vi "Load Alarm Tags and Descriptions.vi"(11 "Alarm Tag Description path":path) -> (2 "Alarm Descriptions":string[](array[string]), 3 "Alarm Array":T1[](array[typedef]))   [LabVIEW 2019]
uses:
  <userlib>/TAE/_SubVIs/TypeDefs/tae_AlarmTagConfiguration.ctl
  <vilib>/NI/Current Value Table/Compatibility/_SubVIs/TypeDefs/cvt_Data Types.ctl
  <userlib>/TAE/_SubVIs/TypeDefs/tae_AlarmConfiguration.ctl
  <userlib>/TAE/_SubVIs/TypeDefs/tae_AlarmType.ctl
  63bfb582-3dd8-4a27-9cf4-6b72469f749e.vi
  <vilib>/Array/Sort 2D Array - Pop Stack.vi
  <vilib>/Array/Sort 2D Array - Push Stack.vi
  <vilib>/Utility/file.llb/Read Delimited Spreadsheet (string).vi
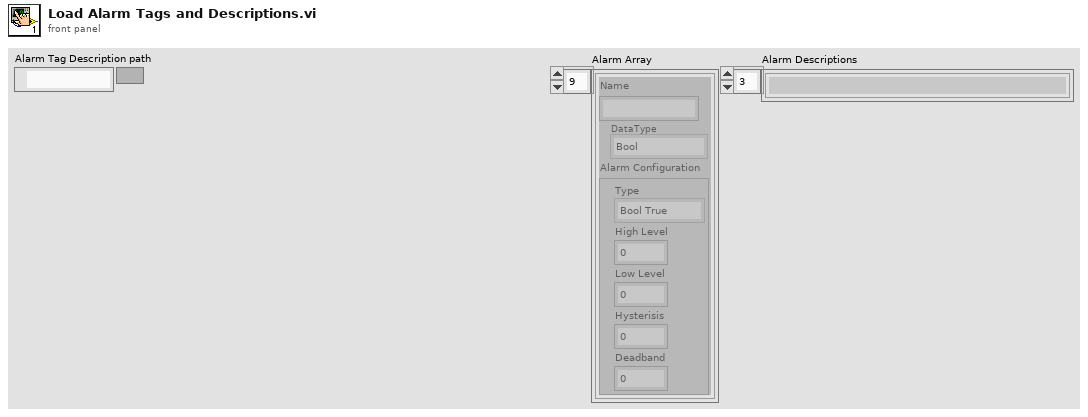
[diagram p1: front panel]
types:
  T1 = typedef "tae_AlarmTagConfiguration.ctl" = cluster{"Name":string, "DataType":T2, "Alarm Configuration":T3}
  T2 = typedef "cvt_Data Types.ctl" = enum16{"Bool", "U8", "I32", "Double", "String", "Enum"}
  T3 = typedef "tae_AlarmConfiguration.ctl" = cluster{"Type":T4, "High Level":dbl, "Low Level":dbl, "Hysterisis":dbl, "Deadband":dbl}
  T4 = typedef "tae_AlarmType.ctl" = enum32{"Bool True", "Bool False", "Over Limit", "Under Limit", "Out-of-Range", "Enum Equal", "Enum Not Equal"}
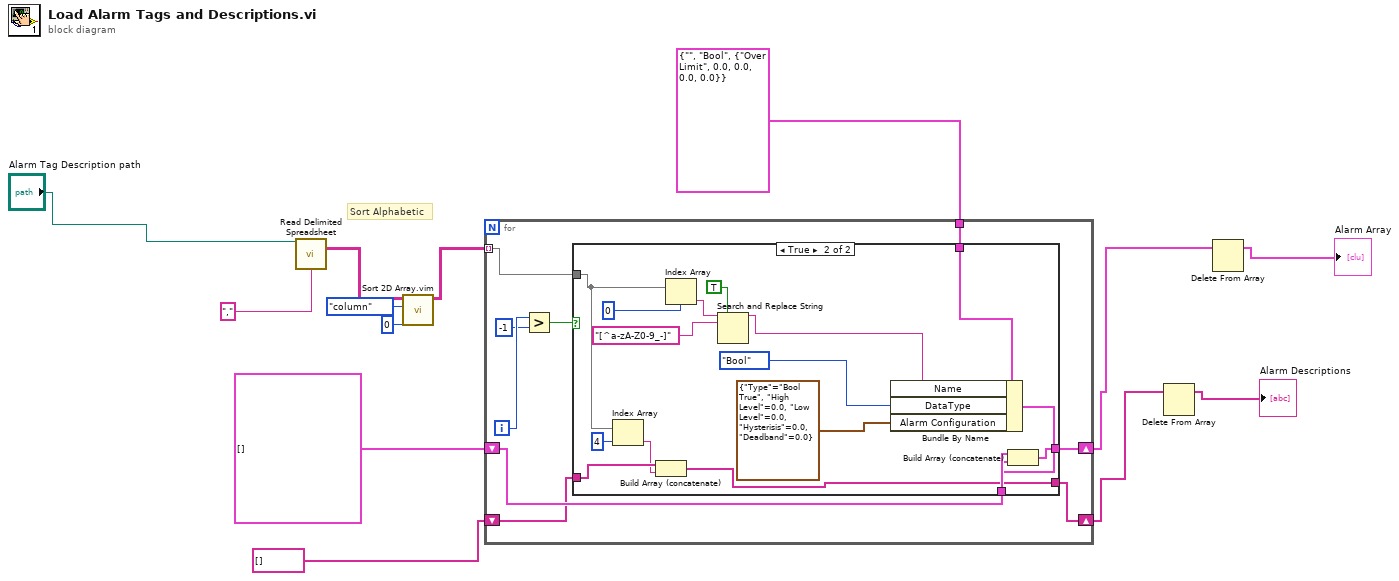
[diagram p0: block diagram]
diagram:
  # "Sort Alphabetic"
  n1 = call-poly <vilib>:"Read Delimited Spreadsheet.vi"("file path (dialog if empty)"="Alarm Tag Description path", "delimiter (\\t)"="," ("delimiter (\\t)")) -> ("all rows"=w9:string[][])  [unwired: 8 in, 5 out]
  n2 = call "Sort 2D Array.vim"("index"=0, "dimension to index (column)"=enum16{"column", "row"}."column", "2D array"=w9) -> ("sorted 2D array"=w6:string[][])  [unwired: 7 in, 1 out]
  n3 = for {
    tunnel: w6 -> [w19] mode=indexing
    tunnel: T1 {"Name"="", "DataType"=enum."Bool", "Alarm Configuration"={"Type"=enum."Over Limit", "High Level"=0.0, "Low Level"=0.0, "Hysterisis"=0.0, "Deadband"=0.0}} ("Alarm List") -> [w18]
    shift-right: [w16] -> w5
    shift-left: T1[] [] ("Alarm Array") -> [w17]
    shift-right: [w14] -> w3
    shift-left: string[] [] ("Alarm Descriptions") -> [w15]
    i -> [w21]
    n4 = Greater?(x=w21, y=-1) -> (0:w22:bool)
    n5 = case shown="True" w22 {
      tunnel: w19 -> [_ w39]
      tunnel: w18 -> [_ w37]
      tunnel: w17 -> [w24 w34]
      tunnel: [w24 w32] -> w16
      tunnel: w15 -> [w23 w31]
      tunnel: [w23 w29] -> w14
      frame False {
      }
      frame True {
        n6 = Index Array(array=w39, index=4) -> (element=w30:string)
        n7 = Build Array (concatenate)(w31, w30) -> (w29:string[])
        n8 = Index Array(array=w39, index=0) -> (element=w28:string)
        n9 = Search and Replace String(replace all?=TRUE ("replace all? (F)"), input string=w28, search string="[^a-zA-Z0-9_-]") -> (result string=w26:string)  [unwired: 5 in, 3 out]
        n10 = Bundle By Name(cluster=w37, "Name"=w26, "DataType"=cvt_Data_Types."Bool", "Alarm Configuration"=T3 {"Type"=enum."Bool True", "High Level"=0.0, "Low Level"=0.0, "Hysterisis"=0.0, "Deadband"=0.0}) -> (w33:T1)
        n11 = Build Array (concatenate)(w34, w33) -> (w32:T1[])
      }
    }
  }
  n12 = Delete From Array(array=w3) -> (array with subset deleted=→"Alarm Descriptions":string[])  [unwired: 2 in, 1 out]
  n13 = Delete From Array(array=w5) -> (array with subset deleted=→"Alarm Array":T1[])  [unwired: 2 in, 1 out]
